vi "Check_Traverse_move_PN.vi"(0 "Current position":sgl[](array[numeric])=[0.0, 0.0, 0.0] format="%.2f", 1 "Traverse Name":string, 2 "Full Check":bool, 5 "New Position":sgl[](array[numeric])=[0.0, 0.0, 0.0] format="%.2f", 7 "Model       Roll      Pitch       Yaw (deg)":sgl[](array[numeric]) format="%#.2f") -> (6 "Position At Crash":dbl[](array[numeric]) format="%.2f", 10 "Steps":sgl[][](array[numeric]) format="%.2f", 15 "Error Comments":string)   [LabVIEW 2014]
uses:
  Collision_Detection/Triangles/EnFlo specific/Collision Mode.ctl
panel:
  # "X                Y                   Z"
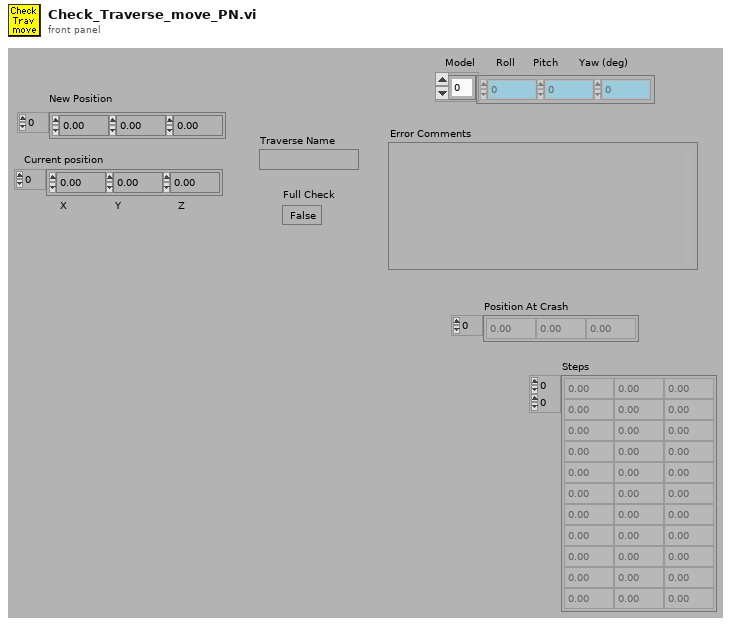
[diagram p1: front panel]
types:
  T1 = enum16{"To Traverse Coordinates", "To User Coordinates"}
  T2 = typedef "Collision Mode.ctl" = enum16{"Traverse - Tunnel", "Traverse - Model", "Traverse - Traverse", "Traverse - All"}
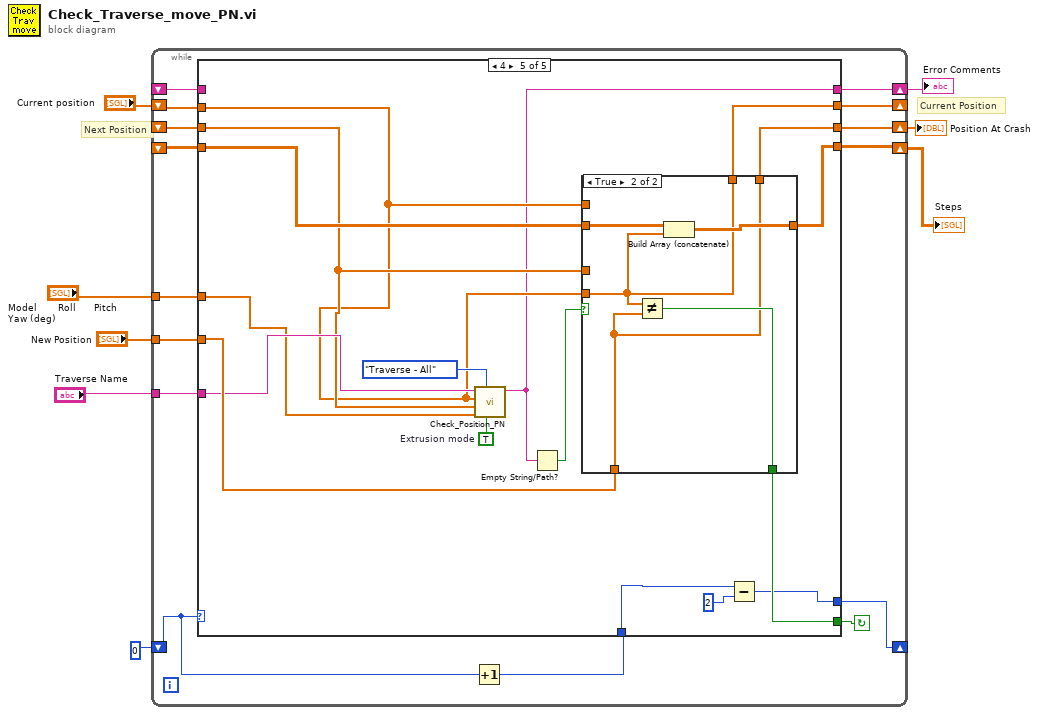
[diagram p0: block diagram]
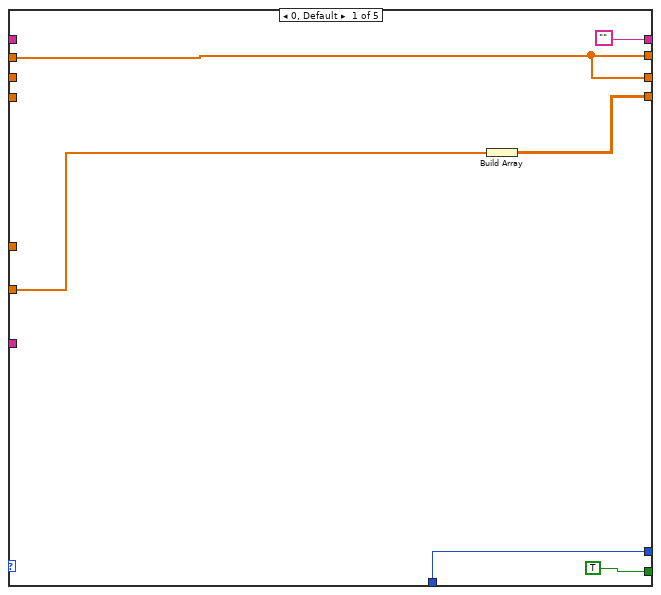
[diagram p2: hidden frame]
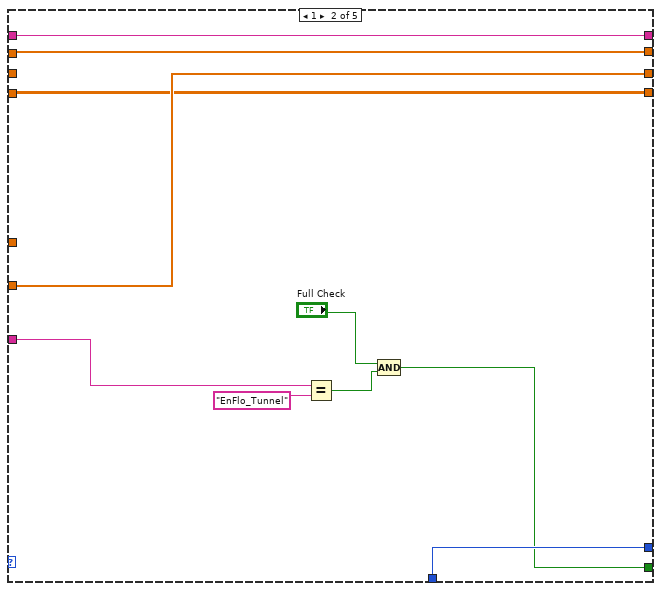
[diagram p3: hidden frame]
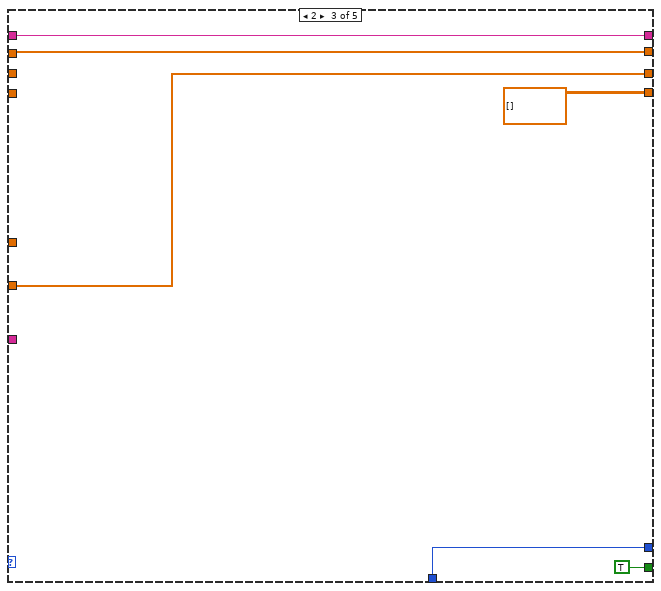
[diagram p4: hidden frame]
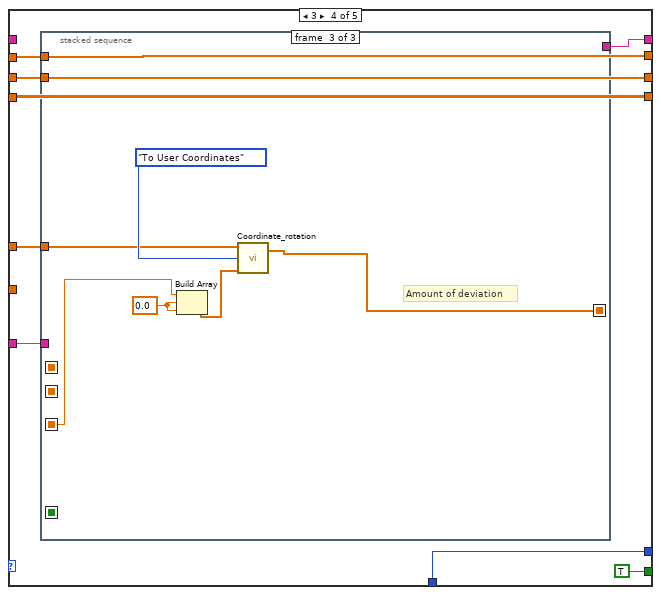
[diagram p5: hidden frame]
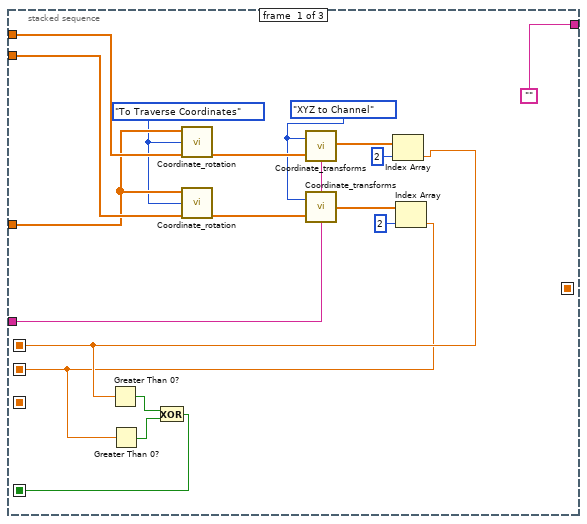
[diagram p6: hidden frame]
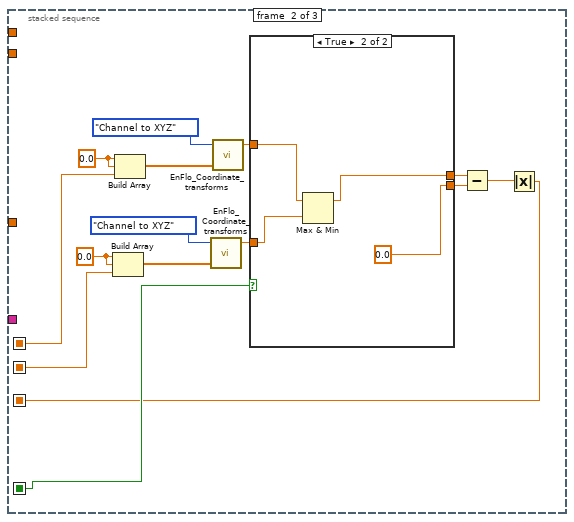
[diagram p7: hidden frame]
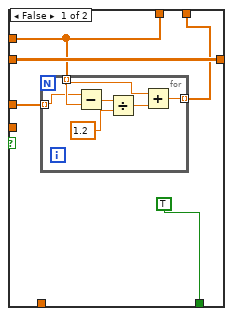
[diagram p9: hidden frame]
diagram:
  # "Current Position"
  # "Next Position"
  n1 = while {
    shift-left: _ -> [w10]
    shift-right: [w9] -> w2
    tunnel: "Model       Roll      Pitch       Yaw (deg)" -> [w11]
    tunnel: "New Position" -> [w12]
    shift-left: _ -> [w14]
    shift-right: [w15] -> w5
    shift-left: 0 -> [w18]
    shift-right: [w17] -> _
    tunnel: "Traverse Name" -> [w19]
    shift-left: _ -> [w13]
    shift-right: [w21] -> w3
    shift-left: "Current position" -> [w23]
    shift-right: [w22] -> _
    stop <- w20 continue-if-true
    n2 = Increment(x=w18) -> (x+1=w16:i32)
    n3 = case shown="4" w18 {
      tunnel: w23 -> [w24 w38 w44 w51 w100]
      tunnel: [w24 w38 w44 w51 w110] -> w22
      tunnel: [w24 w32 w42 w50 w109] -> w21
      tunnel: [TRUE ("Box Inside") w34 TRUE ("Box Inside") TRUE ("Box Inside") w111] -> w20
      tunnel: w19 -> [_ w35 _ w48 w103]
      tunnel: [w26 w37 w43 w47 w107] -> w17
      tunnel: w16 -> [w26 w37 w43 w47 w106]
      tunnel: ["" w39 w45 w53 w99] -> w15
      tunnel: w14 -> [_ w39 w45 _ _]
      tunnel: w13 -> [_ _ _ w50 w102]
      tunnel: w12 -> [w29 w32 w42 _ w112]
      tunnel: w11 -> [_ _ _ w49 w101]
      tunnel: w10 -> [_ w31 _ w46 w115]
      tunnel: [w28 w31 dbl[][] [] w46 w114] -> w9
      frame 0, Default {
        n4 = Build Array(w29) -> (w28:sgl[][])
      }
      frame 1 {
        n5 = Equal?(x=w35, y="EnFlo_Tunnel") -> (x = y?=w30:bool)
        n6 = Compound Arithmetic op=AND("Full Check", w30) -> (w34:bool)
      }
      frame 2 {
      }
      frame 3 {
        n7 = stacked-sequence {
          seq-local: [w56 _ _] -> [_ w86 _]
          seq-local: [w55 _ _] -> [_ w85 _]
          seq-local: [w54 _ _] -> [_ w76 _]
          seq-local: [_ w72 _] -> [_ _ w95]
          seq-local: [_ _ w93] -> [_ _ _]
          tunnel: ["" _ _] -> w53
          tunnel: w51 -> [w69 _ _]
          tunnel: w50 -> [w67 _ _]
          tunnel: w49 -> [w66 _ w94]
          tunnel: w48 -> [w65 _ _]
          frame #0 {
            w63 = enum16{"XYZ to Channel", "Channel to XYZ"}."XYZ to Channel" ("Mode")
            w64 = T1."To Traverse Coordinates" ("Mode")
            n8 = call "Coordinate_rotation.vi"("Model       Roll      Pitch       Yaw (deg)"=w66, "Input Position"=w69, "Mode"=w64) -> ("Output Position"=w70:sgl[])  [unwired: 2 in, 1 out]
            n9 = call "Coordinate_rotation.vi"("Model       Roll      Pitch       Yaw (deg)"=w66, "Input Position"=w67, "Mode"=w64) -> ("Output Position"=w68:sgl[])  [unwired: 2 in, 1 out]
            n10 = call "Coordinate_transforms.vi"("Traverse Name"=w65, "Input"=w70, "Mode"=w63) -> ("Output"=w62:sgl[])
            n11 = call "Coordinate_transforms.vi"("Traverse Name"=w65, "Input"=w68, "Mode"=w63) -> ("Output"=w59:sgl[])
            n12 = Index Array(array=w62, index=2) -> (element=w56:sgl)
            n13 = Greater Than 0?(x=w56) -> (x > 0?=w58:bool)
            n14 = Index Array(array=w59, index=2) -> (element=w55:sgl)
            n15 = Greater Than 0?(x=w55) -> (x > 0?=w57:bool)
            n16 = Exclusive Or(1:w57, 2:w58) -> (0:w54:bool)
          }
          frame #1 {
            w79 = 0.0 ("element")
            w84 = 0.0 ("element")
            n17 = Build Array(w79, w79, w85) -> (w81:dbl[])
            n18 = Build Array(w84, w84, w86) -> (w82:dbl[])
            n19 = call "EnFlo_Coordinate_transforms.vi"("Input"=w81, "Mode"=enum16{"XYZ to Channel", "Channel to XYZ"}."Channel to XYZ") -> ("X theta"=w77:dbl)  [unwired: 3 out]
            n20 = call "EnFlo_Coordinate_transforms.vi"("Input"=w82, "Mode"=enum16{"XYZ to Channel", "Channel to XYZ"}."Channel to XYZ") -> ("X theta"=w78:dbl)  [unwired: 3 out]
            n21 = case shown="True" w76 {
              tunnel: w78 -> [w88 w91]
              tunnel: w77 -> [w87 w92]
              tunnel: [w87 0.0 ("element")] -> w75
              tunnel: [w88 w90] -> w74
              frame False {
              }
              frame True {
                n22 = Max & Min(x=w91, y=w92) -> (max(x,y)=w90:dbl)  [unwired: 1 out]
              }
            }
            n23 = Subtract(x=w74, y=w75) -> (x-y=w73:dbl)
            n24 = Absolute Value(x=w73) -> (abs(x)=w72:dbl)
          }
          frame #2 {
            w97 = 0.0 ("Input Element")
            # "Amount of deviation"
            n25 = Build Array(w95, w97, w97) -> (w96:dbl[])
            n26 = call "Coordinate_rotation.vi"("Model       Roll      Pitch       Yaw (deg)"=w94, "Input Position"=w96, "Mode"=T1."To User Coordinates") -> ("Output Position"=w93:sgl[])  [unwired: 2 in, 1 out]
          }
        }
      }
      frame 4 {
        w104 = TRUE  # Extrusion mode
        n27 = call "Check_Position_PN.vi"("Extrusion mode"=w104, "Collision mode"=Collision_Mode."Traverse - All", "Model Rotation (deg)"=w101, "Traverse extruded position"=w102, "Position to check"=w100, "Traverse Name"=w103) -> ("Error Comments"=w99:string)  [unwired: 2 in, 1 out]
        n28 = Empty String/Path?(string/path=w99) -> (empty?=w113:bool)
        n29 = case shown="True" w113 {
          tunnel: w115 -> [w120 w131]
          tunnel: w100 -> [_ w128]
          tunnel: [w120 w130] -> w114
          tunnel: w112 -> [_ w127]
          tunnel: [TRUE w129] -> w111
          tunnel: [w118 w128] -> w110
          tunnel: [w116 w127] -> w109
          tunnel: w100 -> [w118 _]
          tunnel: w102 -> [w117 _]
          frame False {
            n30 = for {
              tunnel: w118 -> [w122] mode=indexing
              tunnel: w117 -> [w121] mode=indexing
              tunnel: [w123] -> w116 mode=indexing
              n31 = Subtract(x=w121, y=w122) -> (x-y=w126:dbl)
              n32 = Divide(x=w126, y=1.2) -> (x/y=w124:dbl)
              n33 = Add(x=w122, y=w124) -> (x+y=w123:dbl)
            }
          }
          frame True {
            n34 = Not Equal?(x=w128, y=w127) -> (x != y?=w129:bool)
            n35 = Build Array (concatenate)(w131, w128) -> (w130:dbl[][])
          }
        }
        n36 = Subtract(x=w106, y=2) -> (x-y=w107:i32)
      }
    }
  }
  "Error Comments" <- w5
  "Position At Crash" <- w3
  "Steps" <- w2
